vi "Read Output Map.vi"(8 "error in (no error)":errorcluster, 11 "SystemLink runtime in":refnum<class "SystemLink runtime.lvclass">) -> (0 "error out":errorcluster, 2 "Output":T1[](array[typedef]), 3 "SystemLink runtime out":refnum<class "SystemLink runtime.lvclass">)   [LabVIEW 2015, in "SystemLink runtime.lvclass"]
uses:
  SystemLink runtime.lvclass
  configuration/SysLink Mapping.ctl
  <vilib>/Skyline/Tag/Wrapper/Wrapper_class/NI Skyline Tag.lvclass
  configuration/Data Tag Type.ctl
  SystemLink runtime.lvclass/SystemLink runtime.ctl
  configuration/SystemLink configuration.lvclass
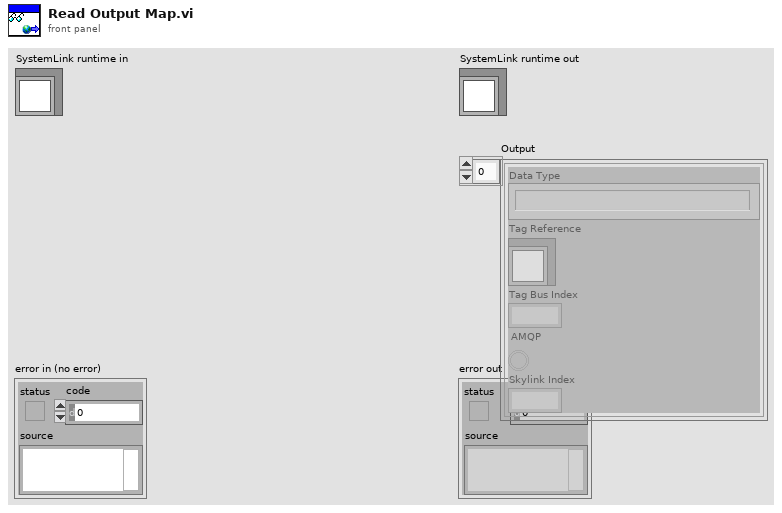
[diagram p1: front panel]
types:
  T1 = typedef "SystemLink configuration.lvclass/SysLink Mapping.ctl" = cluster{"Data Type":T2, "Tag Reference":refnum<class "NI Skyline Tag.lvclass">, "Tag Bus Index":i32, "AMQP":bool, "Skylink Index":i32}
  T2 = typedef "SystemLink configuration.lvclass/Data Tag Type.ctl" = enum16{"Double", "Single", "I32", "I16", "I8", "U64", "U32", "U16", "U8", "Boolean", "String", "Timestamp"}
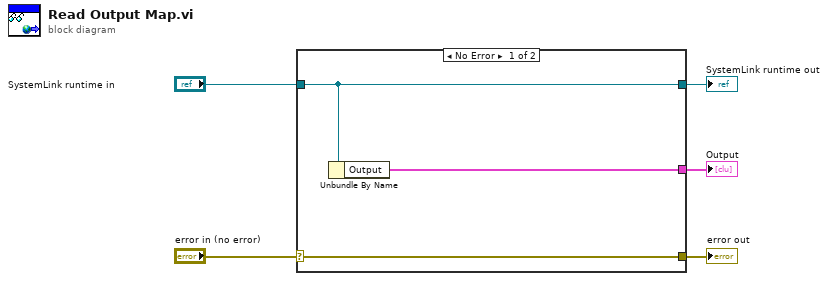
[diagram p0: block diagram]
diagram:
  n1 = case shown="No Error" "error in (no error)" {
    selector: "error in (no error)" -> [w8 w9]
    tunnel: [w8 w9] -> w4
    tunnel: [w7 w10] -> w2
    tunnel: "SystemLink runtime in" -> [w7 w10]
    tunnel: [w6 _] -> w1
    frame No Error {
      n2 = Unbundle By Name(w7) -> ("Output"=w6:T1[])
    }
    frame Error {
    }
  }
  "error out" <- w4
  "SystemLink runtime out" <- w2
  "Output" <- w1
